vi "SSL.vi"(0 "System no.":i32=1 min=1 max=4 step=1, 2 "Affected axes":string[](array[string]), 3 "Soft limit mode":bool[](array[boolean]), 5 "error in":errorcluster, 6 "Without axis ID?":bool) -> (19 "error out":errorcluster)   [LabVIEW 2020]
doc: "Sets soft limits on or off (set by NLM.vi and PLM.vi) for specified axes. If Without axis ID is TRUE, then Affected axes is ignored and first field of Soft limit mode array is used.\n\nC-702: Without axis ID = FALSE\nC-844: Without axis ID = FALSE\nC-848: Without axis ID = FALSE\nC-880: Without axis ID = FALSE\nE-755: Without axis ID = FALSE. Command not available for E-755.101.\nC-886: Without axis ID = FALSE. \nC-887, F-206, M-8X0: Without axis ID = FALSE."
panel:
  # "Sets softlimits on or off (set by NLM.vi and PLM.vi) for specified\naxes.  If \"Without axis ID\" is TRUE, then \"Affected axes\" \nis ignored and first field of \"Soft limit mode\" array is used."
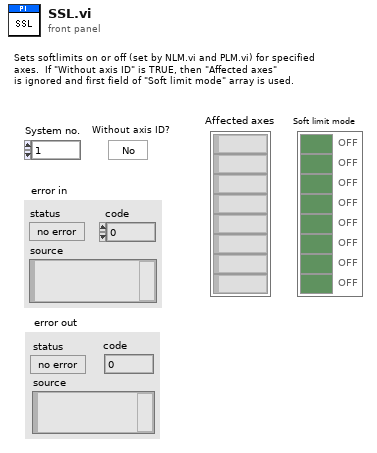
[diagram p1: front panel]
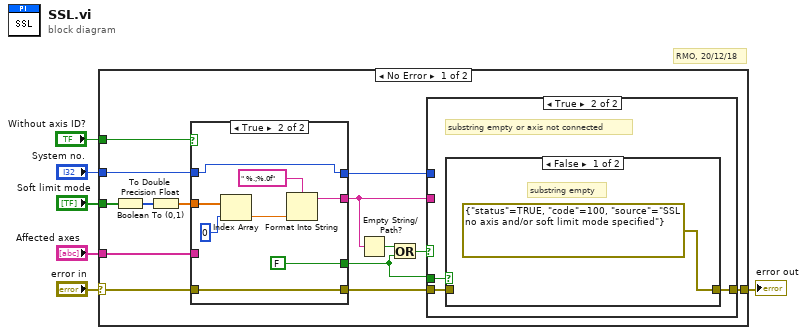
[diagram p0: block diagram]
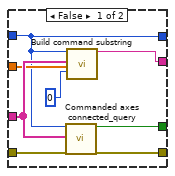
[diagram p2: hidden frame]
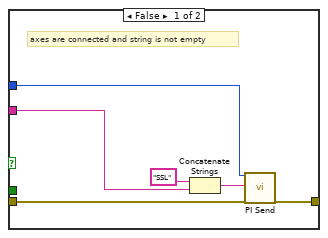
[diagram p3: hidden frame]
diagram:
  # "RMO, 20/12/18"
  n1 = case shown="No Error" "error in" {
    selector: "error in" -> [w13 w48]
    tunnel: [w20 w48] -> w6
    tunnel: "System no." -> [w8 _]
    tunnel: "Affected axes" -> [w18 _]
    tunnel: "Soft limit mode" -> [w17 _]
    tunnel: "Without axis ID?" -> [w14 _]
    frame No Error {
      n2 = Boolean To (0,1)(Boolean=w17) -> (0, 1=w16:i16[])
      n3 = To Double Precision Float(number=w16) -> (double precision float=w15:dbl[])
      n4 = case shown="True" w14 {
        tunnel: [w28 w29] -> w12
        tunnel: w13 -> [w27 w36]
        tunnel: [w26 w36] -> w19
        tunnel: w18 -> [w25 _]
        tunnel: [w24 FALSE] -> w9
        tunnel: w15 -> [w22 w33]
        tunnel: w8 -> [w21 w30]
        tunnel: [w21 w30] -> w7
        frame False {
          n5 = call "Commanded axes connected_query.vi"("System no."=w21, "Commanded axes"=w25, "error in"=w27) -> ("Controller error"=w24:bool, "error out"=w26:errorcluster)  [unwired: 1 in, 14 out]
          n6 = call "Build command substring.vi"("System no."=w21, "Affected axes"=w25, "Parameters"=w22, "No. of digits"=i16 0 ("No.of digits")) -> ("Command substring"=w28:string)  [unwired: 3 in, 12 out]
        }
        frame True {
          n7 = Index Array(array=w33, index=0 ("Index")) -> (element=w32:dbl)
          n8 = Format Into String(format string=" %.;%.0f" ("Format String"), w32) -> (resulting string=w29:string)  [unwired: 2 in, 1 out]
        }
      }
      n9 = Empty String/Path?(string/path=w12) -> (empty?=w11:bool)
      n10 = Or(x=w11, y=w9) -> (x .or. y?=w10:bool)
      n11 = case shown="True" w10 {
        tunnel: w12 -> [w41 _]
        tunnel: [w38 w45] -> w20
        tunnel: w19 -> [w39 w43]
        tunnel: w9 -> [_ w44]
        tunnel: w7 -> [w37 _]
        frame False {
          # "axes are connected and string is not empty"
          n12 = Concatenate Strings("SSL", w41) -> (w40:string)
          n13 = call "PI Send.vi"("System no."=w37, "String to send"=w40, "error in"=w39) -> ("error out"=w38:errorcluster)  [unwired: 3 in, 13 out]
        }
        frame True {
          # "substring empty or axis not connected"
          n14 = case shown="False" w44 {
            tunnel: [errorcluster {"status"=TRUE, "code"=100, "source"="SSL no axis and/or soft limit mode specified"} ("error out") w47] -> w45
            tunnel: w43 -> [_ w47]
            frame False {
              # "substring empty"
            }
            frame True {
              # "commanded axis not connected"
            }
          }
        }
      }
    }
    frame Error {
    }
  }
  "error out" <- w6
